vi "startup.vi"(8 "error in (no error)":errorcluster {"code" format="Error %.0f"}, 10 "Device IDN":string) -> (0 "error out":errorcluster {"code" format="Error %.0f"}, 3 "messageQueues":T4, 4 "SubViRefs":T1, 5 "Notifiers":T3, 7 "userEvents":T2)   [LabVIEW 2017]
uses:
  Message Queues/messageQueues.ctl
  Message Queues/Message Cluster.ctl
  Notifiers/notifiers.ctl
  User Events/userEvents.ctl
  Controls/objectRefsMain.ctl
  User Events/sendRefs.ctl
  Controls/SubViRefs.ctl
  Message Queues/Message Queue.lvlib
  User Events/User Event - Stop.lvlib
  Notifiers/notifiers.lvlib
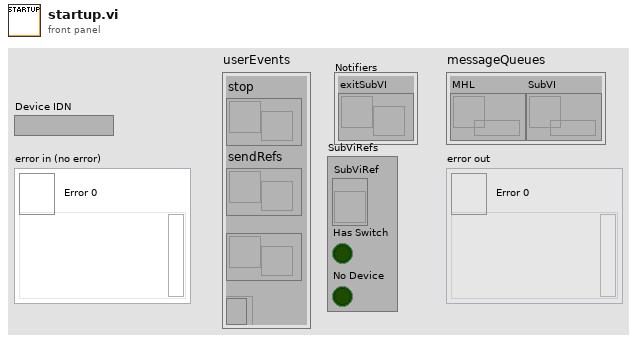
[diagram p1: front panel]
types:
  T1 = typedef "SubViRefs.ctl" = cluster{"SubViRef":refnum<vi>, "Has Switch":bool, "No Device":bool}
  T2 = typedef "User Event - Stop.lvlib/userEvents.ctl" = cluster{"stop":refnum<user-event>, "sendRefs":refnum<user-event>, "sendSubVIRefs":refnum<user-event>, "eventRegRef":refnum<event-registration>}
  T3 = typedef "notifiers.lvlib/notifiers.ctl" = cluster{"exitSubVI":refnum<notifier>}
  T4 = typedef "Message Queue.lvlib/messageQueues.ctl" = cluster{"MHL":refnum<queue>, "SubVI":refnum<queue>}
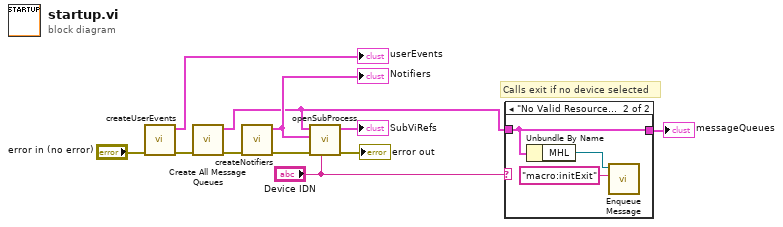
[diagram p0: block diagram]
diagram:
  # "Calls exit if no device selected"
  n1 = call "createUserEvents.vi"("error in (no error)"="error in (no error)") -> ("error out"=w11:errorcluster, "userEvents"=→"userEvents":T2)  [unwired: 9 in]
  n2 = call "Create All Message Queues.vi"("error in (no error)"=w11) -> ("error out"=w9:errorcluster, "messageQueuesOut"=w2:T4)  [unwired: 9 in]
  n3 = call "createNotifiers.vi"("error in"=w9) -> ("error out"=w8:errorcluster, "notifiers"=w7:T3)  [unwired: 9 in]
  "Notifiers" <- w7
  n4 = call "openSubProcess.vi"("Device IDN"="Device IDN", "error in (no error)"=w8, "notifiers"=w7, "messageQueues"=w2) -> ("error out"=→"error out":errorcluster, "SubViRefsOut"=→"SubViRefs":T1)  [unwired: 6 in]
  n5 = case shown="\"No Valid Resource\"" "Device IDN" {
    tunnel: w2 -> [w12 w13]
    tunnel: [w12 w13] -> w3
    frame Default {
    }
    frame "No Valid Resource" {
      n6 = Unbundle By Name(w13) -> ("MHL"=w14:refnum<queue>)
      n7 = call "Enqueue Message.vi"("Message"="macro:initExit", "Message Queue"=w14) -> ()  [unwired: 8 in, 2 out]
    }
  }
  "messageQueues" <- w3
